vi "TW_Thing-Split.vi"(11 "Property":string) -> (0 "Property":string, 3 "Thing":string)   [LabVIEW 2020]
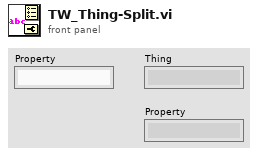
[diagram p1: front panel]
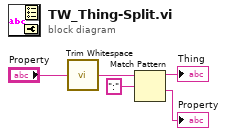
[diagram p0: block diagram]
diagram:
  n1 = call <vilib>:"Trim Whitespace.vi"("string"="Property") -> ("trimmed string"=w5:string)  [unwired: 1 in]
  n2 = Match Pattern(string=w5, regular expression=":") -> (before substring=→"Thing":string, after substring=→"Property":string)  [unwired: 1 in, 2 out]
